vi "Protocol.Create XNET Sessions.vi"(8 "error in (no error)":errorcluster, 11 "Parameters in":T6={"Name"="", "XNET.Settings"={"Database"="", "Cluster"="", "Port"="", "Baud rate [Bd]"=0, "Termination"=0, "Incoming Decimation"=0, "Outgoing Decimation"=1}, "Monitor.Network"={"Address"=0, "Name"=0, "Include DA"=FALSE}, "Data"=[], "DTCs"=[], "Sim.Nodes.LUT"=variant, "Data.LUT"=variant, "PCL"=0} {"Monitor.Network"."Name" format="%.0x"; "DTCs"."Data"."DM1.Ref"."Data Reference" format="%.0x"; "DTCs"."Data"."DM1.Enable.Ref"."Data Reference" format="%.0x"; "DTCs"."Data"."DM2.Ref"."Data Reference" format="%.0x"; "DTCs"."Data"."DM2.Enable.Ref"."Data Reference" format="%.0x"; "Data"."Trigger.Refs"."Data Reference" format="%.0x"; "Data"."Disable.Refs"."Data Reference" format="%.0x"; "Data"."Timing.Refs"."Data Reference" format="%.0x"; "Data"."Network"."Name" format="%.0x"; "Data"."Incoming.Refs"."Data Reference" format="%.0x"; "Data"."Outgoing.Refs"."Data Reference" format="%.0x"; "XNET.Settings"."Termination" items=["Off", "On"]}) -> (0 "error out":errorcluster, 2 "Stream Refs":T1 {"Port Settings"."FD ISO Mode" items=["ISO", "Non ISO", "ISO Legacy"]; "Port Settings"."Termination" items=["Off", "On"]; "Port Settings"."Mode" items=["CAN 2.0", "CAN FD", "CAN FD+BRS"]}, 3 "XNET":T24)   [LabVIEW 2019, in "J1939 Addon Engine.lvlib"]
uses:
  J1939 Addon Engine.lvlib
  <resource>/objmgr/xnet.rc
  Types/Protocol.XNET Settings.ctl
  <vilib>/xnet/xnet.llb/XNET Control Scope.ctl
  <vilib>/xnet/xnet.llb/XNET Create Session (Frame Input Stream).vi
  SubModules/CAN-Streaming-Support/Source/Addon/Addon Engine/CAN Stream Support Engine.lvlib
  <vilib>/xnet/xnet.llb/XNET Create Session (Frame Output Stream).vi
  SubModules/CAN-Streaming-Support/Source/Addon/Addon Engine/Types/Engine Stream Port Settings.ctl
  Addon Shared/Types/XNET Settings.ctl
  Addon Shared/J1939 Addon Shared.lvlib
  <vilib>/NI VeriStand/Custom Device API/Data Reference.ctl
  <vilib>/NI VeriStand/Custom Device API/Custom Device API.lvlib
  <vilib>/NI VeriStand/Custom Device API/Block Data Reference.ctl
  Addon Shared/Types/Monitor Settings.ctl
  Types/Protocol.XNET Refs.ctl
  Types/Engine.DTC FIFOs.ctl
  Addon Shared/Types/Compiled Simulated Settings.ctl
  Types/Engine.DTC Settings.ctl
  Types/Protocol.App Settings.ctl
  Types/Main.Outgoing.Frame.Settings.ctl
  Addon Shared/Types/Outgoing Event Trigger Types.ctl
  SubModules/Frame-Protection-Support/Source/Shared/Types/Exported Frame Settings.ctl
  SubModules/Frame-Protection-Support/Source/Shared/Protection and Counter Support Shared.lvlib
  SubModules/Frame-Protection-Support/Source/Shared/Types/Exported Counter Settings.ctl
  SubModules/Frame-Protection-Support/Source/Shared/Types/XNET Signal Configuration.ctl
  SubModules/Frame-Protection-Support/Source/Shared/Types/Protection Type.ctl
  SubModules/Frame-Protection-Support/Source/Shared/Types/Exported Protection Settings.ctl
  SubModules/Frame-Protection-Support/Source/Shared/Types/Exported Event Trigger Type.ctl
  SubModules/Frame-Protection-Support/Source/Shared/Types/Exported Frame Type.ctl
  SubModules/CAN-Streaming-Support/Source/Addon/Addon Shared/Types/Type Filter.ctl
  SubModules/CAN-Streaming-Support/Source/Addon/Addon Shared/CAN Stream Support Shared.lvlib
  SubModules/CAN-Streaming-Support/Source/Addon/Addon Shared/Types/Direction Filter.ctl
  SubModules/CAN-Streaming-Support/Source/Addon/Addon Shared/Types/Filter Parameters.ctl
  SubModules/CAN-Streaming-Support/Source/Addon/Addon Engine/Types/Engine Stream Refs.ctl
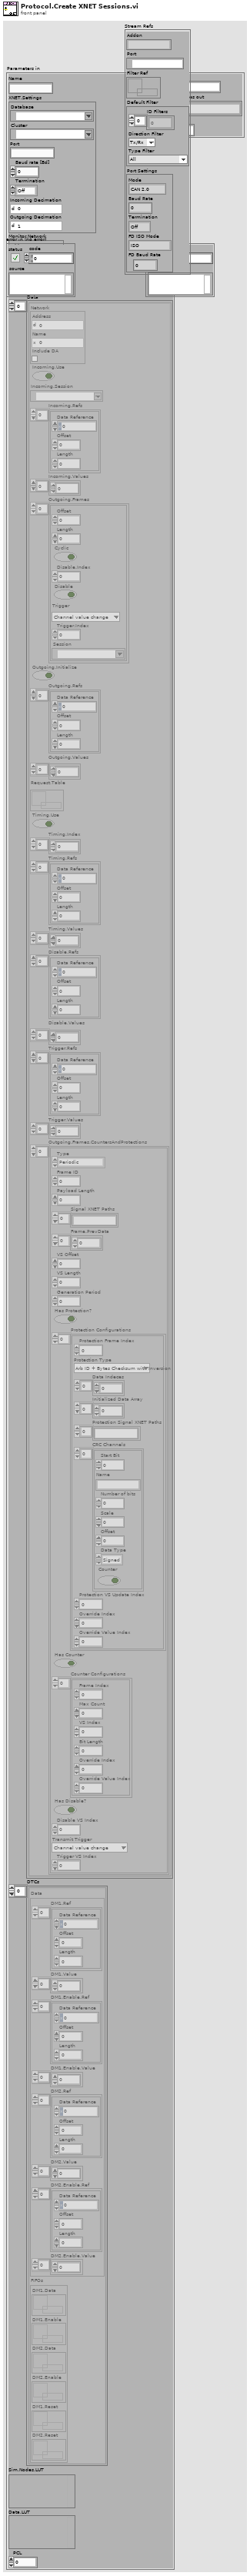
[diagram p1: front panel]
types:
  T1 = typedef "CAN Stream Support Engine.lvlib/Engine Stream Refs.ctl" = cluster{"Addon":string, "Port":refnum<k21>, "Filter Ref":refnum<data-value>, "Default Filter":T2, "Port Settings":T5}
  T2 = typedef "CAN Stream Support Shared.lvlib/Filter Parameters.ctl" = cluster{"ID Filters":u32[], "Direction Filter":T3, "Type Filter":T4}
  T3 = typedef "CAN Stream Support Shared.lvlib/Direction Filter.ctl" = enum16{"Tx/Rx", "Rx", "Tx"}
  T4 = typedef "CAN Stream Support Shared.lvlib/Type Filter.ctl" = enum16{"All", "CAN Data", "CAN Remote", "CAN Bus Error", "CAN 2.0 Data", "CAN FD Data", "CAN FD+BRS Data", "J1939 Data", "Delay", "Log Trigger", "Start Trigger"}
  T5 = typedef "CAN Stream Support Engine.lvlib/Engine Stream Port Settings.ctl" = cluster{"Mode":u32, "Baud Rate":u64, "Termination":u32, "FD ISO Mode":u32, "FD Baud Rate":u64}
  T6 = typedef "J1939 Addon Engine.lvlib/Protocol.App Settings.ctl" = cluster{"Name":string, "XNET.Settings":T7, "Monitor.Network":T8, "Data":T9[], "DTCs":T21[], "Sim.Nodes.LUT":variant, "Data.LUT":variant, "PCL":u32}
  T7 = typedef "J1939 Addon Shared.lvlib/XNET Settings.ctl" = cluster{"Database":refnum<k21>, "Cluster":refnum<k21>, "Port":string, "Baud rate [Bd]":u32, "Termination":u32, "Incoming Decimation":u32, "Outgoing Decimation":u32}
  T8 = typedef "J1939 Addon Shared.lvlib/Monitor Settings.ctl" = cluster{"Address":u8, "Name":u64, "Include DA":bool}
  T9 = typedef "J1939 Addon Engine.lvlib/Protocol.XNET Refs.ctl" = cluster{"Network":T8, "Incoming.Use":bool, "Incoming.Session":refnum<k21>, "Incoming.Refs":T10[], "Incoming.Values":dbl[], "Outgoing.Frames":T12[], "Outgoing.Initialize":bool, "Outgoing.Refs":T10[], "Outgoing.Values":dbl[], "Request.Table":refnum<k33>, "Timing.Use":bool, "Timing.Index":i32[], "Timing.Refs":T10[], "Timing.Values":dbl[], "Disable.Refs":T10[], "Disable.Values":dbl[], "Trigger.Refs":T10[], "Trigger.Values":dbl[], "Outgoing.Frames.CountersAndProtections":T14[]}
  T10 = typedef "Custom Device API.lvlib/Block Data Reference.ctl" = cluster{"Data Reference":T11, "Offset":u64, "Length":u64}
  T11 = typedef "Custom Device API.lvlib/Data Reference.ctl" = i32
  T12 = typedef "J1939 Addon Engine.lvlib/Main.Outgoing.Frame.Settings.ctl" = cluster{"Offset":u32, "Length":u32, "Cyclic":bool, "Disable.Index":i32, "Disable":bool, "Trigger":T13, "Trigger.Index":i32, "Session":refnum<k21>}
  T13 = typedef "J1939 Addon Shared.lvlib/Outgoing Event Trigger Types.ctl" = enum16{"Channel value change", "Trigger channel (not zero)", "Channel value change or trigger channel (not zero)", "Trigger channel (any value change)", "Channel value change or trigger channel (any value change)"}
  T14 = typedef "Protection and Counter Support Shared.lvlib/Exported Frame Settings.ctl" = cluster{"Type":T15, "Frame ID":u32, "Payload Length":u32, "Signal XNET Paths":string[], "Frame.PrevData":dbl[], "VS Offset":i32, "VS Length":i32, "Generation Period":u32, "Has Protection?":bool, "Protection Configurations":T16[], "Has Counter":bool, "Counter Configurations":T19[], "Has Disable?":bool, "Disable VS Index":i32, "Transmit Trigger":T20, "Trigger VS Index":i32}
  T15 = typedef "Protection and Counter Support Shared.lvlib/Exported Frame Type.ctl" = enum16{"Periodic", "Event", "Periodic/Event"}
  T16 = typedef "Protection and Counter Support Shared.lvlib/Exported Protection Settings.ctl" = cluster{"Protection Frame Index":i32, "Protection Type":T17, "Data Indeces":i32[], "Initialized Data Array":dbl[], "Protection Signal XNET Paths":string[], "CRC Channels":T18[], "Protection VS Update Index":i32, "Override Index":i32, "Override Value Index":i32}
  T17 = typedef "Protection and Counter Support Shared.lvlib/Protection Type.ctl" = enum16{"Arb ID + Bytes Checksum with Inversion", "Arb ID + Bytes CRC with Inversion", "Reversed Raw Signal Checksum with Inversion", "Concatenated Two's Compliment"}
  T18 = typedef "Protection and Counter Support Shared.lvlib/XNET Signal Configuration.ctl" = cluster{"Start Bit":i32, "Name":string, "Number of bits":i32, "Scale":dbl, "Offset":dbl, "Data Type":u32, "Counter":bool}
  T19 = typedef "Protection and Counter Support Shared.lvlib/Exported Counter Settings.ctl" = cluster{"Frame Index":i32, "Max Count":dbl, "VS Index":i32, "Bit Length":i64, "Override Index":i32, "Override Value Index":i32}
  T20 = typedef "Protection and Counter Support Shared.lvlib/Exported Event Trigger Type.ctl" = enum16{"Channel value change", "Trigger channel (not zero)", "Channel value change or trigger channel (not zero)", "Trigger channel (any value change)", "Channel value change or trigger channel (any value change)"}
  T21 = typedef "J1939 Addon Engine.lvlib/Engine.DTC Settings.ctl" = cluster{"Data":T22, "FIFOs":T23}
  T22 = typedef "J1939 Addon Shared.lvlib/Compiled Simulated Settings.ctl" = cluster{"DM1.Ref":T10[], "DM1.Value":dbl[], "DM1.Enable.Ref":T10[], "DM1.Enable.Value":dbl[], "DM2.Ref":T10[], "DM2.Value":dbl[], "DM2.Enable.Ref":T10[], "DM2.Enable.Value":dbl[]}
  T23 = typedef "J1939 Addon Engine.lvlib/Engine.DTC FIFOs.ctl" = cluster{"DM1.Data":refnum<k33>, "DM1.Enable":refnum<k33>, "DM2.Data":refnum<k33>, "DM2.Enable":refnum<k33>, "DM1.Reset":refnum<k33>, "DM2.Reset":refnum<k33>}
  T24 = typedef "J1939 Addon Engine.lvlib/Protocol.XNET Settings.ctl" = cluster{"Raw CAN In":refnum<k21>, "Raw Frames out":refnum<k21>[], "Raw J1939 In":refnum<k21>}
  T25 = typedef "XNET Control Scope.ctl" = u32
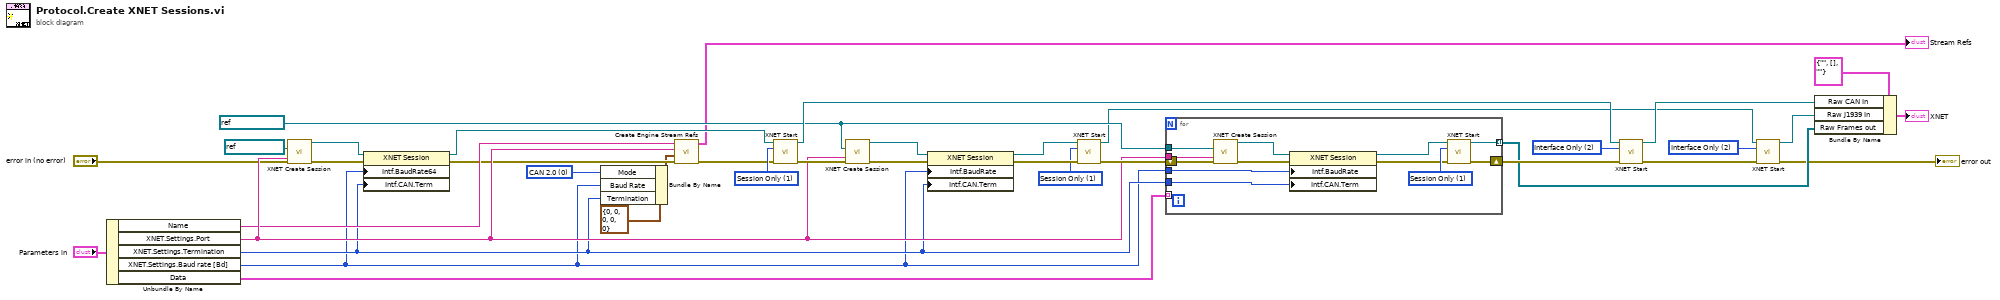
[diagram p0: block diagram]
diagram:
  w3 = u32 0 items=["CAN 2.0", "CAN FD", "CAN FD+BRS"] ("Mode")
  w16 = T25 2 items=["Normal", "Session Only", "Interface Only", "Session Only Blocking"] ("scope (normal)")
  w23 = T25 1 items=["Normal", "Session Only", "Interface Only", "Session Only Blocking"] ("scope (normal)")
  w31 = T25 2 items=["Normal", "Session Only", "Interface Only", "Session Only Blocking"] ("scope (normal)")
  w33 = T25 1 items=["Normal", "Session Only", "Interface Only", "Session Only Blocking"] ("scope (normal)")
  w17 = refnum<k21> ":can_j1939:" ("cluster (:memory:)")
  n1 = Unbundle By Name("Parameters in") -> ("Name"=w10:string, "XNET.Settings.Port"=w11:string, "XNET.Settings.Termination"=w2:u32, "XNET.Settings.Baud rate [Bd]"=w1:u32, "Data"=w27:T9[])
  n2 = call-poly <vilib>:"XNET Create Session.vi"("cluster (:memory:)"=refnum<k21> ":memory:", "interface"=w11, "error in (no error)"="error in (no error)") -> ("session out"=w34:refnum<k21>, "error out"=w35:errorcluster)  [unwired: 11 out]
  n3 = property class="XNET Session"(reference=w34, error in=w35, "Intf.BaudRate64"=w1, "Intf.CAN.Term"=w2) -> (reference out=w32:refnum<k21>, error out=w8:errorcluster)
  n4 = Bundle By Name(cluster=T5 {"Mode"=0, "Baud Rate"=0, "Termination"=0, "FD ISO Mode"=0, "FD Baud Rate"=0} ("Port Settings"), "Mode"=w3, "Baud Rate"=w1, "Termination"=w2) -> (w4:T5)
  n5 = call "Create Engine Stream Refs.vi"("error in (no error)"=w8, "Port Settings"=w4, "Port"=w11, "Addon"=w10) -> ("error out"=w7:errorcluster, "Refs"=→"Stream Refs":T1)  [unwired: 6 in]
  n6 = call <vilib>:"XNET Start.vi"("session in"=w32, "scope (normal)"=w33, "error in (no error)"=w7) -> ("session out"=w29:refnum<k21>, "error out"=w21:errorcluster)  [unwired: 11 in]
  n7 = call-poly <vilib>:"XNET Create Session.vi"("cluster (:memory:)"=w17, "interface"=w11, "error in (no error)"=w21) -> ("session out"=w18:refnum<k21>, "error out"=w22:errorcluster)  [unwired: 11 out]
  n8 = property class="XNET Session"(reference=w18, error in=w22, "Intf.BaudRate"=w1, "Intf.CAN.Term"=w2) -> (reference out=w19:refnum<k21>, error out=w24:errorcluster)
  n9 = call <vilib>:"XNET Start.vi"("session in"=w19, "scope (normal)"=w23, "error in (no error)"=w24) -> ("session out"=w13:refnum<k21>, "error out"=w20:errorcluster)  [unwired: 11 in]
  n10 = for {
    tunnel: [w39] -> w26 mode=indexing
    tunnel: w1 -> [w50]
    tunnel: w2 -> [w49]
    tunnel: w11 -> [w48]
    tunnel: w17 -> [w45]
    shift-right: [w41] -> w30
    shift-left: w20 -> [w44]
    tunnel: w27 -> [_] mode=indexing
    w43 = T25 1 items=["Normal", "Session Only", "Interface Only", "Session Only Blocking"] ("scope (normal)")
    n11 = call-poly <vilib>:"XNET Create Session.vi"("cluster (:memory:)"=w45, "interface"=w48, "error in (no error)"=w44) -> ("session out"=w46:refnum<k21>, "error out"=w47:errorcluster)  [unwired: 11 out]
    n12 = property class="XNET Session"(reference=w46, error in=w47, "Intf.BaudRate"=w50, "Intf.CAN.Term"=w49) -> (reference out=w40:refnum<k21>, error out=w42:errorcluster)
    n13 = call <vilib>:"XNET Start.vi"("session in"=w40, "scope (normal)"=w43, "error in (no error)"=w42) -> ("session out"=w39:refnum<k21>, "error out"=w41:errorcluster)  [unwired: 11 in]
  }
  n14 = call <vilib>:"XNET Start.vi"("session in"=w29, "scope (normal)"=w31, "error in (no error)"=w30) -> ("session out"=w28:refnum<k21>, "error out"=w15:errorcluster)  [unwired: 11 in]
  n15 = call <vilib>:"XNET Start.vi"("session in"=w13, "scope (normal)"=w16, "error in (no error)"=w15) -> ("session out"=w12:refnum<k21>, "error out"=→"error out":errorcluster)  [unwired: 11 in]
  n16 = Bundle By Name(cluster=T24 {"Raw CAN In"="", "Raw Frames out"=[], "Raw J1939 In"=""} ("XNET"), "Raw CAN In"=w28, "Raw J1939 In"=w12, "Raw Frames out"=w26) -> (→"XNET":T24)
